vi "PH_ImageCalibrator.write PixelSum.vi"(0 "i ref in":refnum<vi>, 2 "Cam Image":T1, 5 "error in (no error)":errorcluster) -> (14 "i ref out":refnum<vi>, 19 "error out":errorcluster)   [LabVIEW 2014, in "PH_ImageCalibrator.lvlib"]
doc: "If background and cam image have the same size, this VI subtracts the background image from the cam image, calculates the pixel sum, adds the old value of the pixel sum and writes it to the attributes. In this case it is also set that the background has been subtracted. If no background image of the right size is available, the sum is written to the attribues but the flag is not set.."
uses:
  PH_ImageCalibrator.lvlib
  <vilib>/vision/Image Controls.llb/IMAQ Image.ctl
  <vilib>/vision/NI_Vision_Development_Module.lvlib
  PH_Basics/PH_Image_Common/PH_Image_Common.lvlib
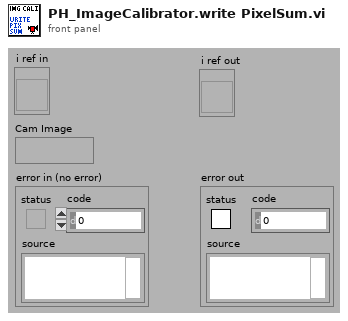
[diagram p1: front panel]
types:
  T1 = typedef "IMAQ Image.ctl" = refnum<image>
  T2 = typedef "PH_ImageCalibrator.lvlib/PH_ImageCalibrator.i attribute.ctl" = cluster{"GUI Refs":cluster{"Available Cams":refnum<vi>, "OK":refnum<vi>, "Skip":refnum<vi>, "Repeat":refnum<vi>, "Cancel":refnum<vi>, "Length [mm]":refnum<vi>, "Energy [mJ]":refnum<vi>, "Dialog":refnum<vi>}, "Cam instances":string[], "Dark Pics":cluster{"#":i32, "BI taken":bool}, "Lin Cali":cluster{"Distance [Pixel]":dbl, "Distance [mm]":dbl, "Lin Cali Factor [mm/Pixel]":dbl}, "Energy Cali":cluster{"Pixelsum":dbl, "Energy [mJ]":dbl, "Energy Cali factor [mJ/Pixelsum]":dbl, "Underground subtracted?":bool, "#":i32}, "Images":cluster{"Background":T1, "Energy":T1}}
  T3 = typedef "Image Type" = u32
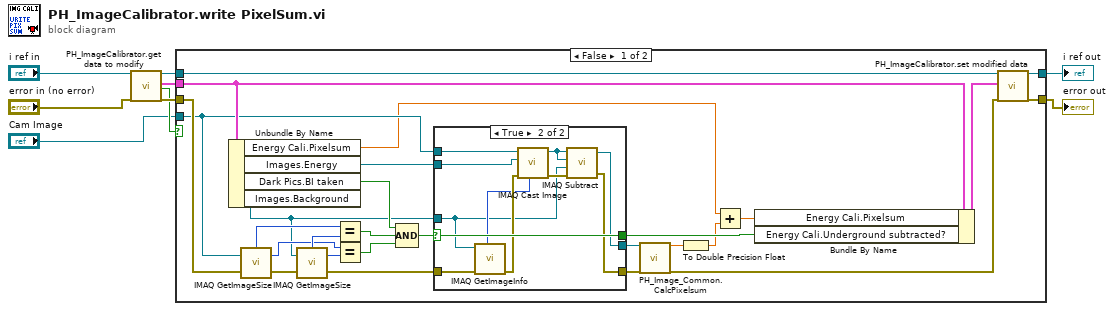
[diagram p0: block diagram]
diagram:
  n1 = call "PH_ImageCalibrator.get data to modify.vi"("i ref in"="i ref in", "error in (no error)"="error in (no error)") -> ("i ref out"=w6:refnum<vi>, "i attribute"=w9:T2, "timed out"=w2:bool, "error out"=w3:errorcluster)  [unwired: 14 in]
  n2 = case shown="False" w2 {
    tunnel: w9 -> [w32 _]
    tunnel: [w35 w52] -> w8
    tunnel: w6 -> [w34 w52]
    tunnel: [w33 w51] -> w4
    tunnel: w3 -> [w29 w51]
    tunnel: "Cam Image" -> [w14 _]
    frame False {
      n3 = Unbundle By Name(w32) -> ("Energy Cali.Pixelsum"=w11:dbl, "Images.Energy"=w20:T1, "Dark Pics.BI taken"=w16:bool, "Images.Background"=w10:T1)
      n4 = call "IMAQ GetImageSize"("Image"=w14, "error in (no error)"=w29) -> ("Y Resolution"=w26:i32, "X Resolution"=w28:i32, "error out"=w30:errorcluster)  [unwired: 2 in]
      n5 = call "IMAQ GetImageSize"("Image"=w10, "error in (no error)"=w30) -> ("Y Resolution"=w25:i32, "X Resolution"=w27:i32, "error out"=w21:errorcluster)  [unwired: 2 in]
      n6 = Equal?(x=w28, y=w27) -> (x = y?=w24:bool)
      n7 = Equal?(x=w26, y=w25) -> (x = y?=w23:bool)
      n8 = Compound Arithmetic op=AND(w16, w24, w23) -> (w22:bool)
      n9 = case shown="True" w22 {
        selector: w22 -> [w39 w50]
        tunnel: w10 -> [_ w42]
        tunnel: w14 -> [w37 w44]
        tunnel: [w39 w50] -> w31
        tunnel: w21 -> [w38 w49]
        tunnel: [w38 w45] -> w17
        tunnel: w20 -> [_ w40]
        tunnel: [w37 w41] -> w19
        frame False {
        }
        frame True {
          n10 = call "IMAQ GetImageInfo"("error in (no error)"=w49, "Image"=w42) -> ("error out"=w48:errorcluster, "Image Type"=w47:T3)  [unwired: 2 in, 6 out]
          n11 = call "IMAQ Cast Image"("Image Type"=w47, "error in (no error)"=w48, "Image Dst"=w40, "Image Src"=w44) -> ("error out"=w46:errorcluster, "Image Dst Out"=w43:T1)  [unwired: 6 in]
          n12 = call "IMAQ Subtract"("Image Src A"=w43, "Image Dst"=w43, "Image Src B"=w42, "error in (no error)"=w46) -> ("Image Dst Out"=w41:T1, "error out"=w45:errorcluster)  [unwired: 3 in]
        }
      }
      n13 = call "PH_Image_Common.CalcPixelsum.vi"("Image"=w19, "error in (no error)"=w17) -> ("Pixel Sum"=w15:sgl, "error out"=w18:errorcluster)  [unwired: 16 in]
      n14 = To Double Precision Float(number=w15) -> (double precision float=w13:dbl)
      n15 = Add(x=w11, y=w13) -> (x+y=w12:dbl)
      n16 = Bundle By Name(cluster=w32, "Energy Cali.Pixelsum"=w12, "Energy Cali.Underground subtracted?"=w31) -> (w36:T2)
      n17 = call "PH_ImageCalibrator.set modified data.vi"("i ref in"=w34, "i attribute"=w36, "error in (no error)"=w18) -> ("i ref out"=w35:refnum<vi>, "error out"=w33:errorcluster)  [unwired: 15 in]
    }
    frame True {
    }
  }
  "i ref out" <- w8
  "error out" <- w4
